vi "BRig_dataExp_DAB_flipLR_opt.vi"() -> (2 "output_DAB_flipLR_opt":i32)   [LabVIEW 2014]
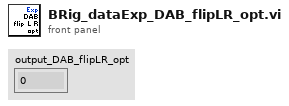
[diagram p1: front panel]
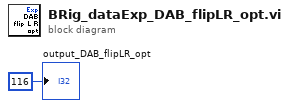
[diagram p0: block diagram]
diagram:
  "output_DAB_flipLR_opt" <- 116 ("output_iBlock")
